vi "rad_Deploy Application Image.vi"(7 "App Image Temp Folder":path=path "C:/dev/Architectures/Reference Designs/Application Deployment and Replication/Application Deployment Utility/trunk/source/Application Images/_temp", 8 "error in (no error)":errorcluster, 10 "Selected Targets":T1[](array[typedef]) {"Primary NIC"."IP Address Request Mode" items=["Static"=1, "DHCP/Link-Local"=2, "Link-Local Only"=4, "DHCP Only"=8]}, 11 "App Image Path":path=path "C:/dev/Architectures/Reference Designs/Application Deployment and Replication/Application Deployment Utility/trunk/source/Application Images/AppImage1.lvappimg") -> (0 "error out":errorcluster, 1 "Cancelled":bool)   [LabVIEW 2023]
uses:
  Targets/TypeDefs/rad_Target Information.ctl
  Targets/TypeDefs/rad_Target Network Settings.ctl
  TypeDefs/rad_Target Configuration Settings.ctl
  TypeDefs/rad_Target Configuration Operations.ctl
  TypeDefs/rad_Deployment Notifiers.ctl
  TypeDefs/rad_Deployment Status Data Type.ctl
  TypeDefs/rad_Deployment Progress Data Type.ctl
  Util/FP Control/FP Control Functions.ctl
  <vilib>/nisyscfg/Close (System).vi
  <vilib>/nisyscfg/nisyscfg.lvlib
panel:
  out "Stop Updates":bool
  in  "Deploy":bool
  in  "Config Options":bool
  in  "Log":bool
  in  "Stop":bool
  in  "State Variables":T6={"App Image Path"=path "C:/dev/Architectures/Reference Designs/Application Deployment and Replication/Application Deployment Utility/trunk/source/Application Images/AppImage1.lvappimg", "App Image Temp Folder"=path "C:/dev/Architectures/Reference Designs/Application Deployment and Replication/Application Deployment Utility/trunk/source/Application Images/_temp", "Targets"=[], "Target Configuration Options"={"NumInBatch"=0, "Target Config Operation"=enum."No Config", "Target Name"="", "Increment Static IPs"=FALSE, "Change Target Name"=FALSE, "Primary NIC"={"MAC address"="", "IP Address Request Mode"=2, "IP address"="", "Subnet mask"="", "Gateway"="", "DNS server"=""}}, "Deployment Notifiers"=[]} {"Target Configuration Options"."Primary NIC"."IP Address Request Mode" items=["Static"=1, "DHCP/Link-Local"=2, "Link-Local Only"=4, "DHCP Only"=8]; "Targets"."Primary NIC"."IP Address Request Mode" items=["Static"=1, "DHCP/Link-Local"=2, "Link-Local Only"=4, "DHCP Only"=8]}
  out "Targets":i32(listbox)
  in  "Close":bool
  # "Targets"
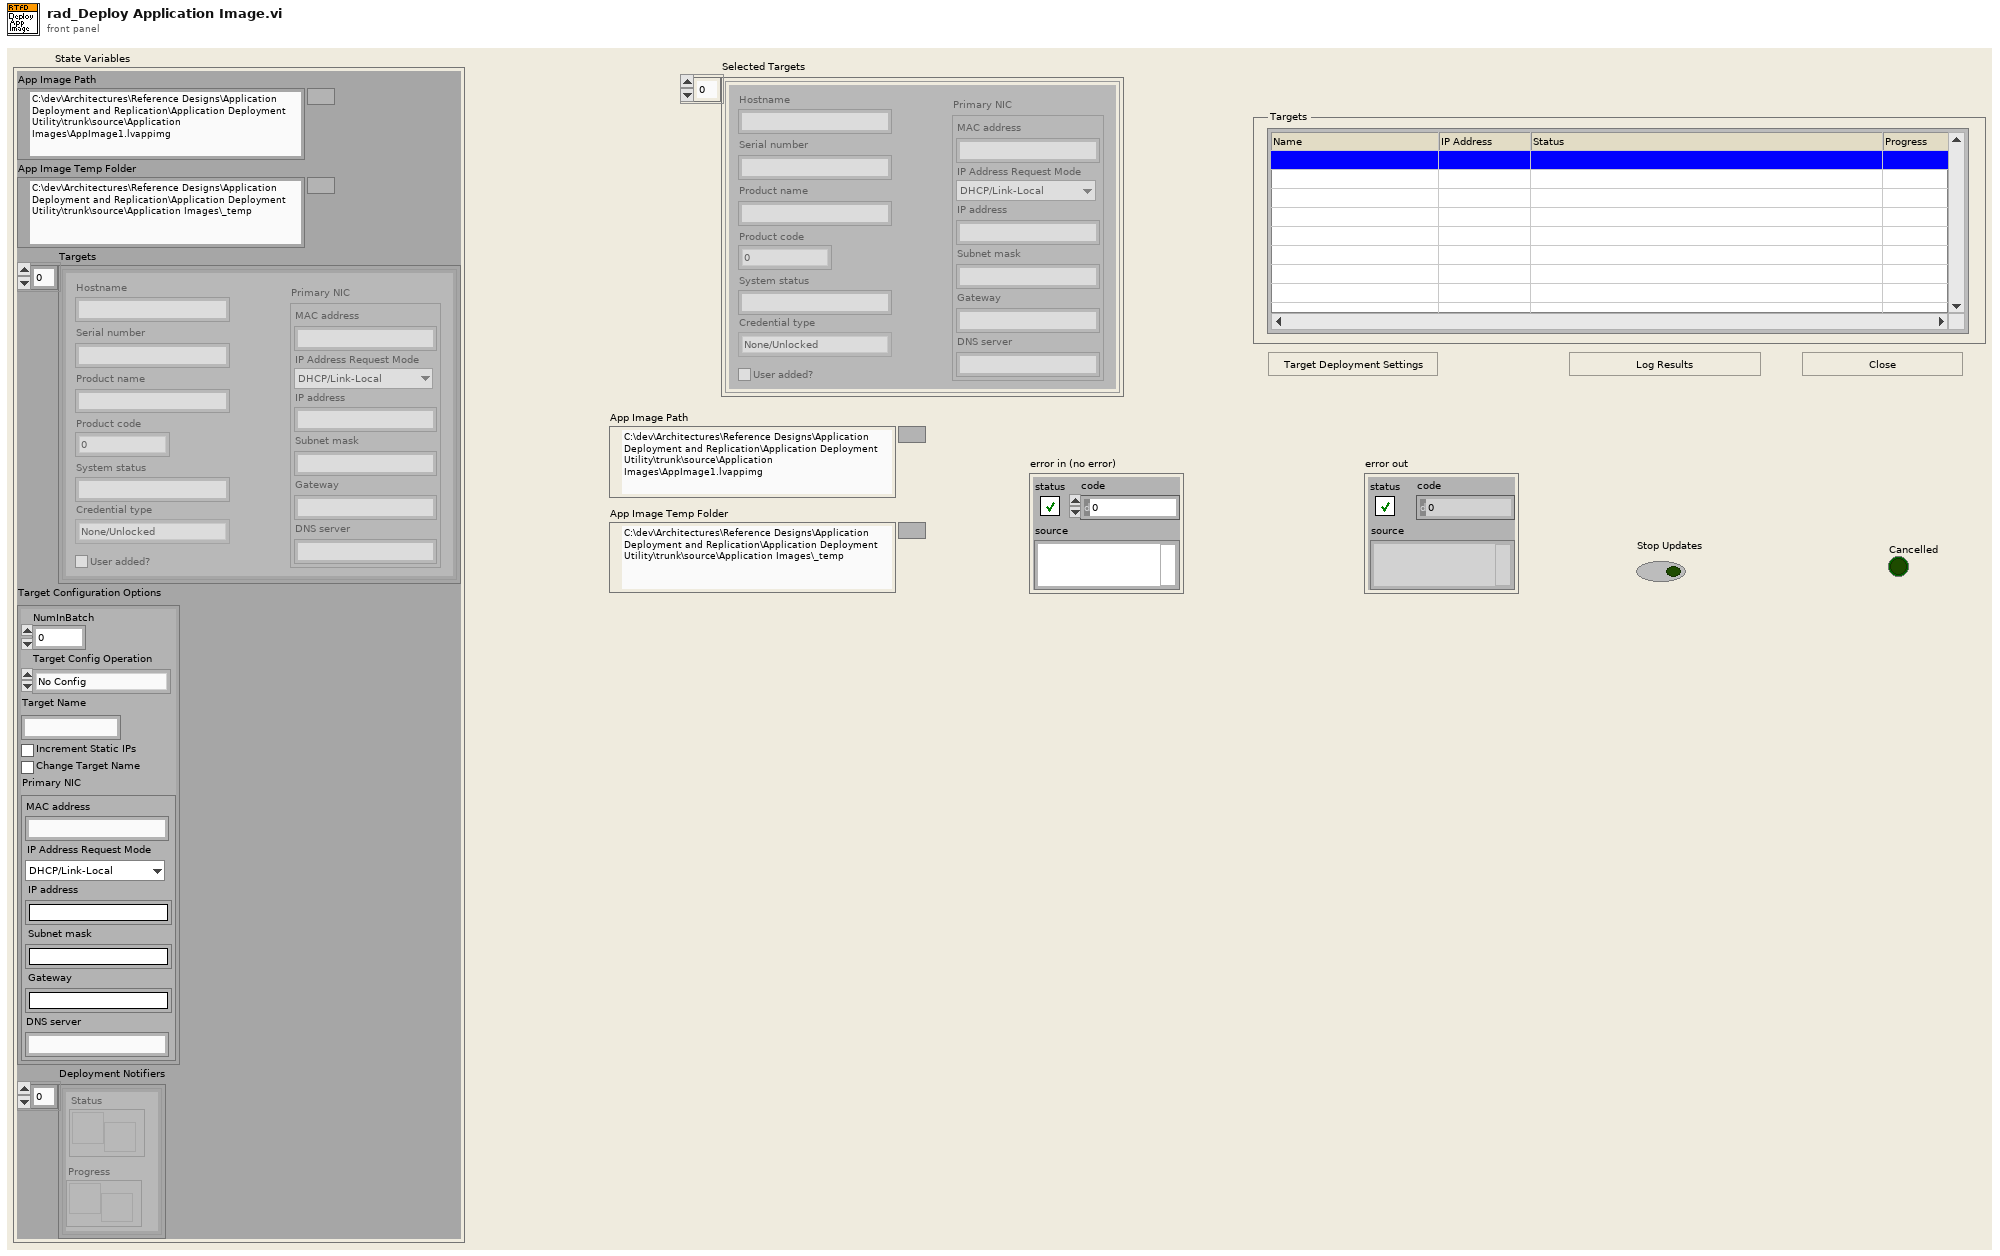
[diagram p1: front panel]
types:
  T1 = typedef "rad_Target Information.ctl" = cluster{"Hostname":string, "Serial number":string, "Product name":string, "Product code":i32, "System status":string, "Credential type":enum16{"None/Unlocked", "FTP Password", "NIAuth Credentials"}, "User added?":bool, "Primary NIC":T2}
  T2 = typedef "rad_Target Network Settings.ctl" = cluster{"MAC address":string, "IP Address Request Mode":i32, "IP address":string, "Subnet mask":string, "Gateway":string, "DNS server":string}
  T3 = typedef "rad_Target Configuration Settings.ctl" = cluster{"NumInBatch":u32, "Target Config Operation":T4, "Target Name":string, "Increment Static IPs":bool, "Change Target Name":bool, "Primary NIC":T2}
  T4 = typedef "rad_Target Configuration Operations.ctl" = enum8{"No Config", "Image Config", "Static Config"}
  T5 = typedef "rad_Deployment Notifiers.ctl" = cluster{"Status":refnum<notifier>, "Progress":refnum<notifier>}
  T6 = cluster{"App Image Path":path, "App Image Temp Folder":path, "Targets":T1[], "Target Configuration Options":T3, "Deployment Notifiers":T5[]}
  T7 = typedef "rad_Deployment Progress Data Type.ctl" = i8
  T8 = typedef "rad_Deployment Status Data Type.ctl" = string
  T9 = typedef "FP Control Functions.ctl" = enum16{"Open", "Close", "Bring To Front", "Center"}
  T10 = enum8{"Enabled", "Disabled", "Disabled and Grayed Out"}
  T11 = typedef "rad_Application Image Properties.ctl" = cluster{"Name":string, "Version":string, "Time":timestamp, "Description":string, "Key":string, "Chassis":string, "FPGA Properties":T12, "Model":string, "Retrieve":string[], "Deploy":string[], "Installed Software":string[]}
  T12 = typedef "rad_FPGA Properties.ctl" = T13[]
  T13 = typedef "rad_FPGA Flash Properties.ctl" = cluster{"Resource Name":string, "Path":path}
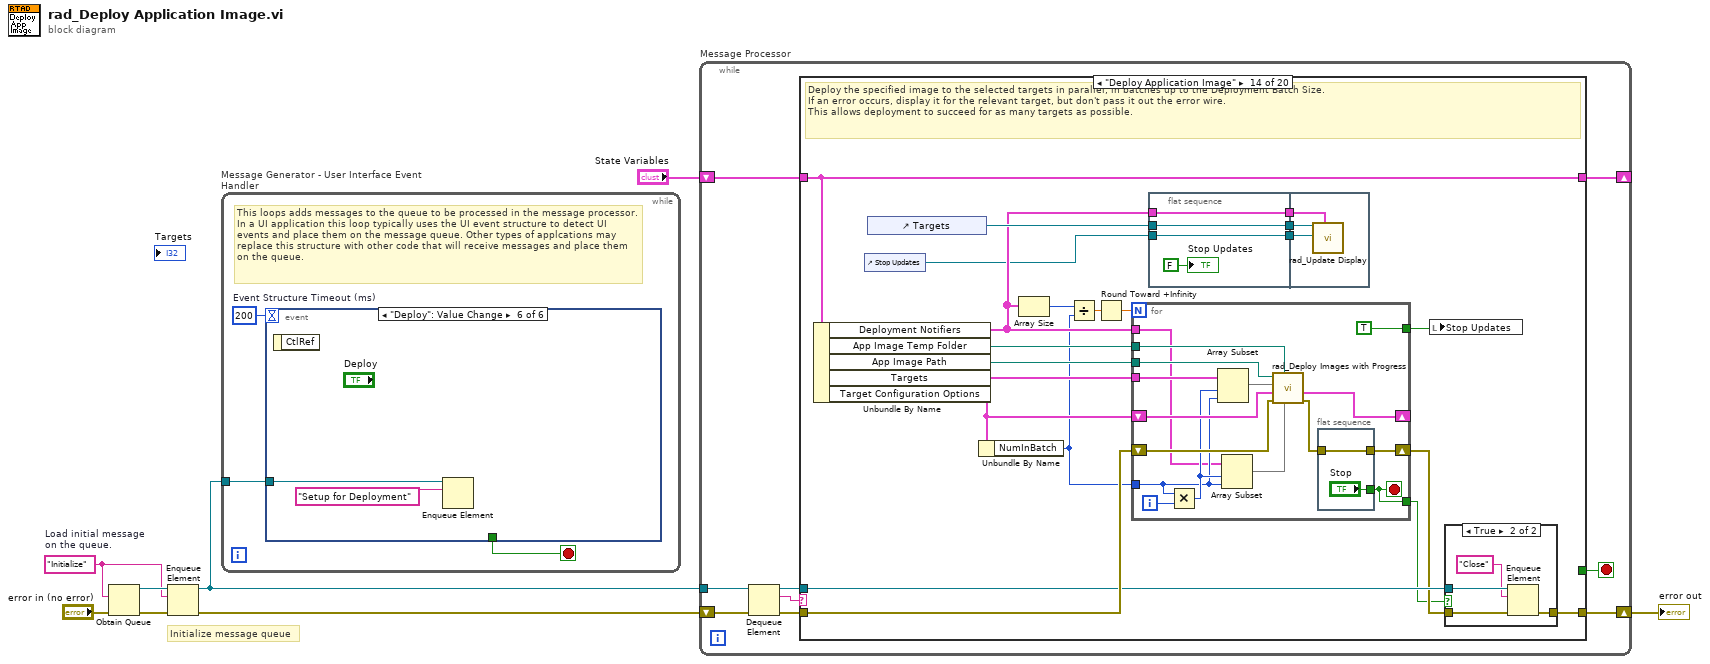
[diagram p0: block diagram]
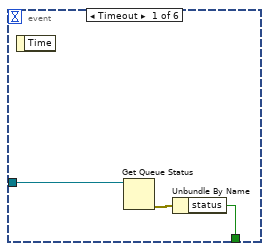
[diagram p2: hidden frame]
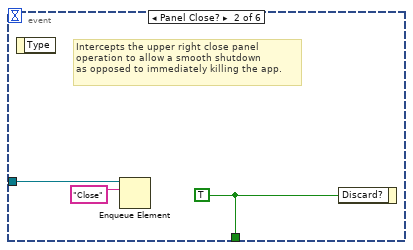
[diagram p3: hidden frame]
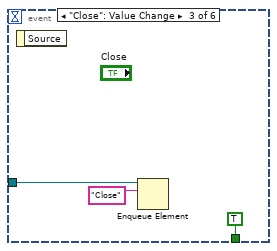
[diagram p4: hidden frame]
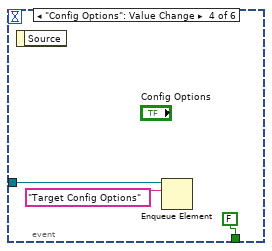
[diagram p5: hidden frame]
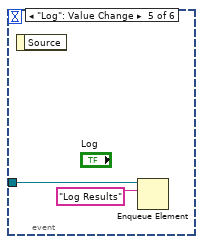
[diagram p6: hidden frame]
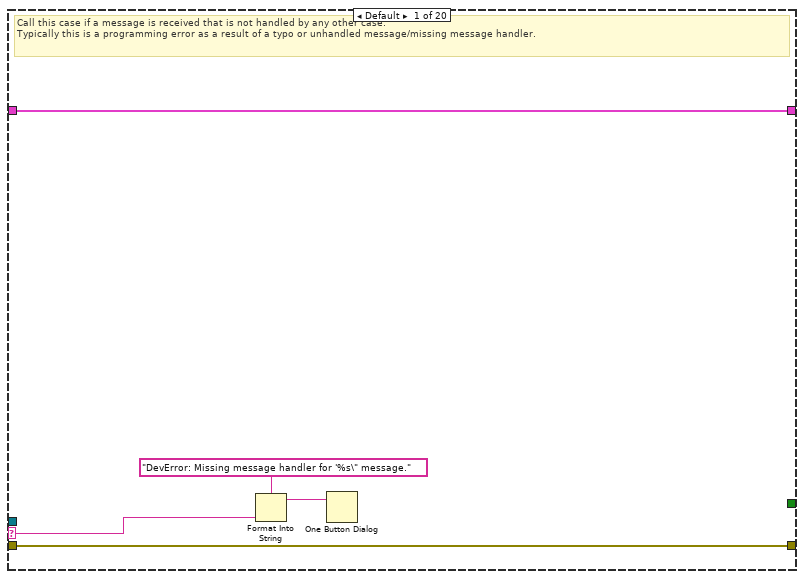
[diagram p7: hidden frame]
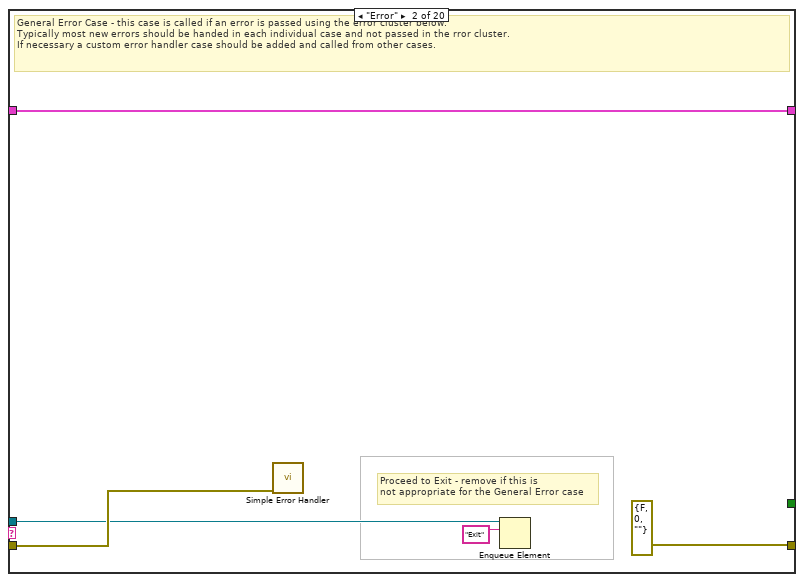
[diagram p8: hidden frame]
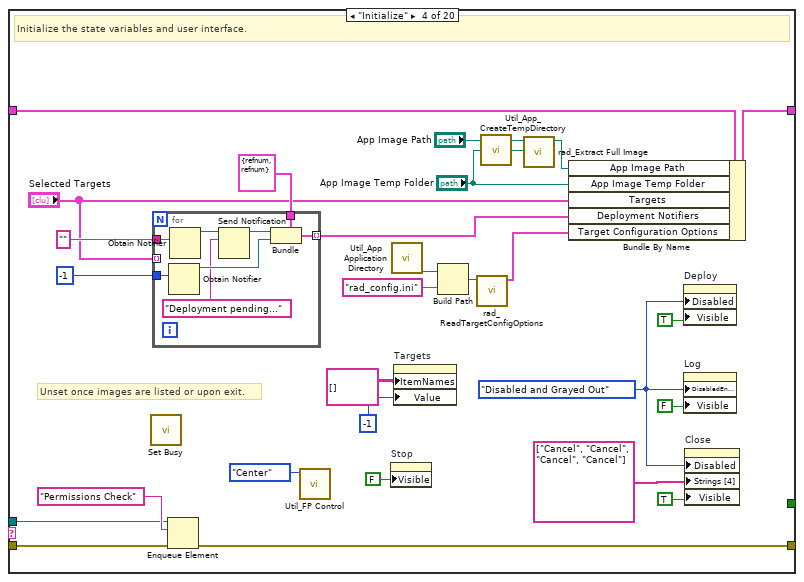
[diagram p10: hidden frame]
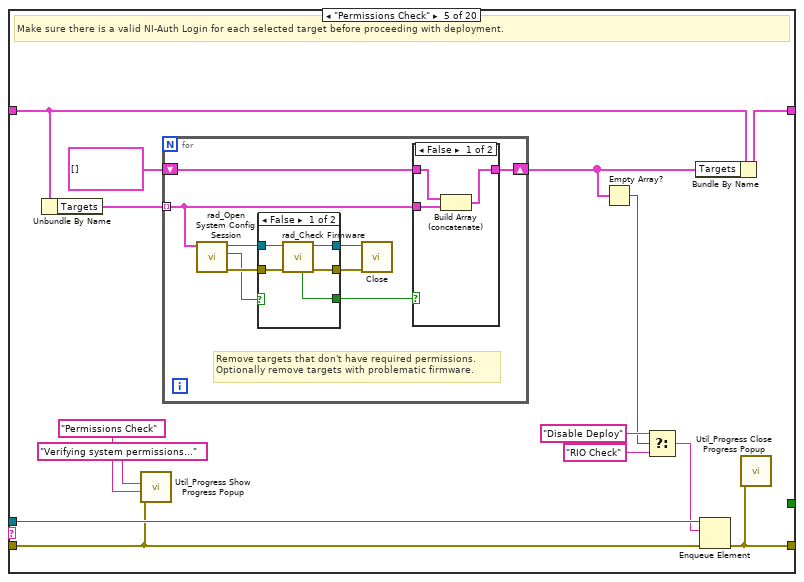
[diagram p11: hidden frame]
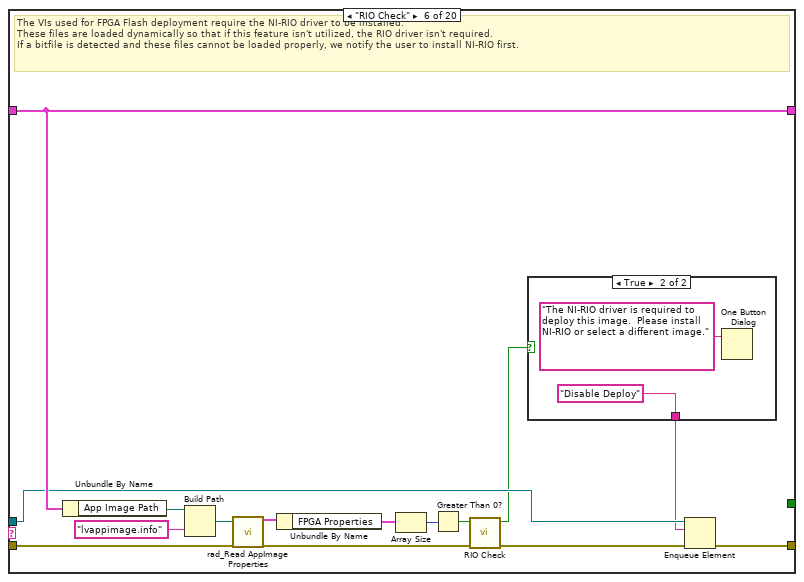
[diagram p14: hidden frame]
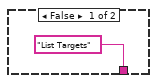
[diagram p15: hidden frame]
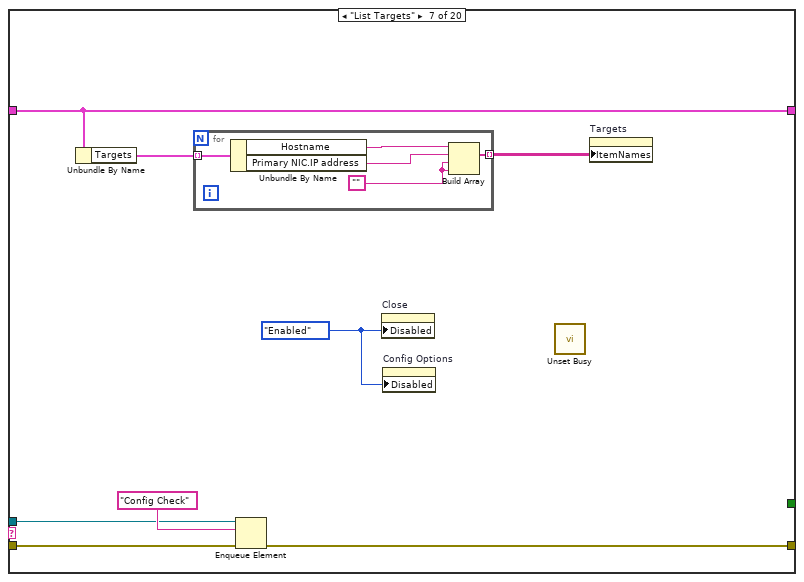
[diagram p16: hidden frame]
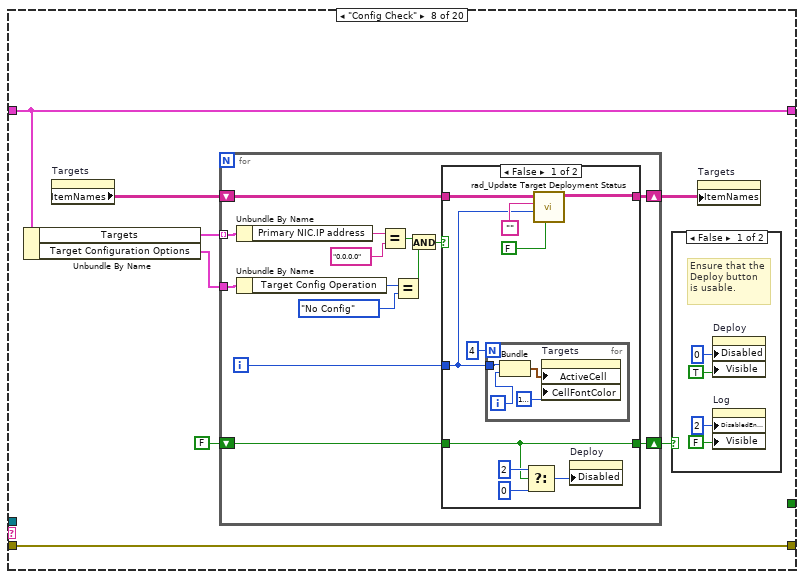
[diagram p17: hidden frame]
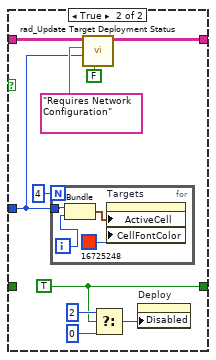
[diagram p19: hidden frame]
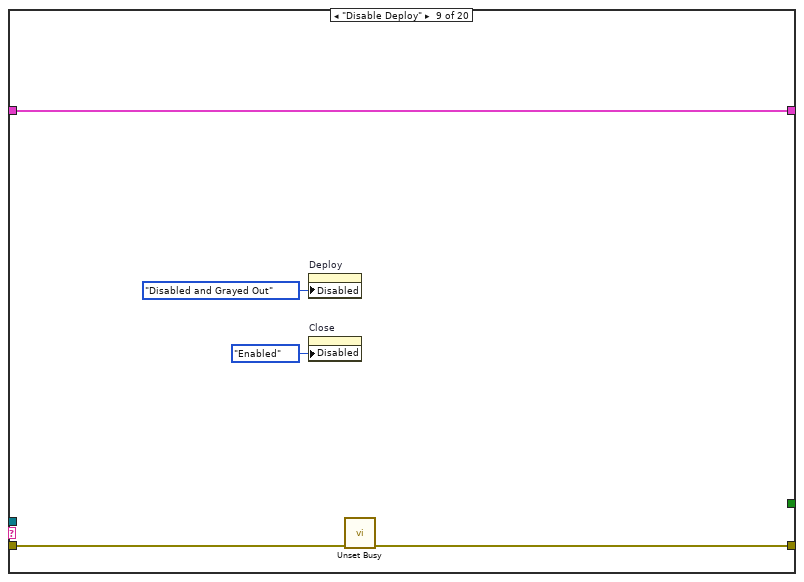
[diagram p20: hidden frame]
diagram:
  w1 = "Initialize"  # Load initial message on the queue.
  # "Initialize message queue"
  n1 = Obtain Queue(element data type=w1, error in (no error)="error in (no error)") -> (queue out=w3:refnum<queue>, error out=w8:errorcluster)  [unwired: 3 in, 1 out]
  n2 = Enqueue Element(queue=w3, element=w1, error in (no error)=w8) -> (queue out=w2:refnum<queue>, error out=w4:errorcluster)  [unwired: 1 in, 1 out]
  n3 = while "Message Generator - User Interface Event Handler" {
    tunnel: w2 -> [w9]
    stop <- w10 stop-if-true
    w11 = 200  # Event Structure Timeout (ms)
    # "This loops adds messages to the queue to be processed in the message processor. In a UI application this loop typically uses the UI event structure to detect UI events and place them on the message queue. Other types of applcations may replace this structure with other code that will receive messages and place them on the queue."
    n4 = event shown="[5] \"Deploy\": Value Change" {
      selector: _ -> [_ _ _ _ _ _]
      dyn-events: _ -> [_ _ _ _ _ _]
      timeout: w11 -> [_ _ _ _ _ _]
      tunnel: [w13 w17 TRUE ("Discard?") FALSE ("Discard?") _ _] -> w10
      tunnel: w9 -> [w12 w16 w20 w23 w25 w27]
      event Timeout {
        n5 = event-data() -> ()  [unwired: 2 out]
        n6 = Get Queue Status(queue=w12) -> (error out=w14:errorcluster)  [unwired: 2 in, 7 out]
        n7 = Unbundle By Name(w14) -> ("status"=w13:bool)
      }
      event Panel Close? {
        w17 = TRUE ("Discard?")
        # "Intercepts the upper right close panel\noperation to allow a smooth shutdown\nas opposed to immediately killing the app."
        n8 = event-data() -> ()  [unwired: 2 out]
        n9 = Enqueue Element(queue=w16, element="Close") -> ()  [unwired: 2 in, 3 out]
        n10 = event-data("Discard?"=w17) -> ()  [unwired: 1 in, 1 out]
      }
      event "Close": Value Change {
        n11 = event-data() -> ()  [unwired: 2 out]
        n12 = Enqueue Element(queue=w20, element="Close") -> ()  [unwired: 2 in, 3 out]
      }
      event "Config Options": Value Change {
        n13 = event-data() -> ()  [unwired: 2 out]
        n14 = Enqueue Element(queue=w23, element="Target Config Options") -> ()  [unwired: 2 in, 3 out]
      }
      event "Log": Value Change {
        n15 = event-data() -> ()  [unwired: 2 out]
        n16 = Enqueue Element(queue=w25, element="Log Results") -> ()  [unwired: 2 in, 3 out]
      }
      event "Deploy": Value Change {
        n17 = event-data() -> ()  [unwired: 2 out]
        n18 = Enqueue Element(queue=w27, element="Setup for Deployment") -> ()  [unwired: 2 in, 3 out]
      }
    }
  }
  n19 = while "Message Processor" {
    shift-left: w4 -> [w31]
    shift-right: [w32] -> w5
    tunnel: w2 -> [w30]
    shift-left: "State Variables" -> [w36]
    shift-right: [w35] -> _
    stop <- w28 stop-if-true
    n20 = Dequeue Element(queue=w30, error in (no error)=w31) -> (queue out=w34:refnum<queue>, element=w29:string, error out=w33:errorcluster)  [unwired: 1 in, 1 out]
    n21 = case shown="\"Deploy Application Image\"" w29 {
      selector: w29 -> [w39 _ _ _ _ _ _ _ _ _ _ _ _ _ _ _ _ _ _ _]
      tunnel: [w41 w46 w48 w75 w95 w131 w143 w153 w207 w211 w213 w219 w239 w258 w295 w303 w305 w313 w316 w323] -> w35
      tunnel: w36 -> [w41 w46 w48 w76 w96 w131 w143 w153 w207 w211 w213 w220 w239 w258 w295 w303 w305 w313 w316 w323]
      tunnel: w34 -> [_ w43 _ w54 w94 w128 w138 _ _ _ _ w217 w235 w253 _ _ _ w307 _ w328]
      tunnel: w33 -> [w40 w44 w47 w70 w90 w123 w140 w158 w209 w210 w212 w221 w240 w257 w296 w301 w304 w308 w314 w329]
      tunnel: [w40 errorcluster {"status"=FALSE, "code"=0, "source"=""} ("error out") w47 w56 w89 w129 w139 w158 w208 w210 w212 w215 w231 w251 w296 w300 w304 w306 w314 w320] -> w32
      tunnel: [_ _ _ _ _ _ _ _ _ _ _ _ _ _ _ _ _ _ _ TRUE] -> w28
      frame Default {
        # "Call this case if a message is received that is not handled by any other case.\nTypically this is a programming error as a result of a typo or unhandled message/missing message handler."
        n22 = Format Into String(format string="DevError: Missing message handler for '%s\" message." ("message"), w39) -> (resulting string=w37:string)  [unwired: 2 in, 1 out]
        n23 = One Button Dialog(message=w37) -> ()  [unwired: 2 out]
      }
      frame "Error" {
        # "Proceed to Exit - remove if this is\nnot appropriate for the General Error case"
        # "General Error Case - this case is called if an error is passed using the error cluster below.\nTypically most new errors should be handed in each individual case and not passed in the rror cluster.\nIf necessary a custom error handler case should be added and called from other cases."
        n24 = call <vilib>:"Simple Error Handler.vi"("error in (no error)"=w44) -> ()  [unwired: 1 in, 8 out]
        n25 = Enqueue Element(queue=w43, element="Exit") -> ()  [unwired: 2 in, 3 out]
      }
      frame "*******Init******" {
        # "Dummy case to add a seperator in the Case Structure menu."
      }
      frame "Initialize" {
        w49 = T10."Disabled and Grayed Out" ("Disabled")
        # "Unset once images are listed or upon exit."
        # "Initialize the state variables and user interface."
        n26 = call <vilib>:"Set Busy.vi"() -> ()  [unwired: 10 in, 2 out]
        n27 = for {
          tunnel: T8 "" ("status notifier data type") -> [w84]
          tunnel: T7 -1 ("Progress") -> [w83]
          tunnel: T5 {"Status"=refnum, "Progress"=refnum} ("Deployment Notifiers") -> [w81]
          tunnel: [w80] -> w65 mode=indexing
          tunnel: "Selected Targets" -> [_] mode=indexing
          n28 = Obtain Notifier(notification data type=w83) -> (notifier out=w82:refnum<notifier>)  [unwired: 3 in, 2 out]
          n29 = Obtain Notifier(notification data type=w84) -> (notifier out=w79:refnum<notifier>)  [unwired: 3 in, 2 out]
          n30 = Send Notification(notification=T8 "Deployment pending...", notifier=w79) -> (notifier out=w78:refnum<notifier>)  [unwired: 1 in, 1 out]
          n31 = Bundle(cluster=w81, "Status"=w78, "Progress"=w82) -> (w80:T5)
        }
        n32 = Enqueue Element(queue=w54, element="Permissions Check", error in (no error)=w70) -> (error out=w56:errorcluster)  [unwired: 1 in, 2 out]
        n33 = call "Util_FP Control.vi"("Function"=FP_Control_Functions."Center") -> ()  [unwired: 1 in, 10 out]
        n34 = property on="Stop" class="Bool"("Visible"=FALSE) -> ()  [unwired: 2 in, 2 out]
        n35 = call "Util_App Application Directory.vi"() -> ("Application Directory"=w64:path)  [unwired: 11 out]
        n36 = property on="Targets" class="MCListbox (strict)"("ItemNames"=string[][] [] ("Item Names"), "Value"=-1 ("Targets")) -> ()  [unwired: 2 in, 2 out]
        n37 = Build Path(base path=w64, name or relative path="rad_config.ini" ("Config File Name")) -> (appended path=w62:path)
        n38 = call "rad_ReadTargetConfigOptions.vi"("configuration file path"=w62) -> ("TargetConfigurationOptions"=w61:T3)  [unwired: 9 in, 1 out]
        n39 = call "Util_App_CreateTempDirectory.vi"("TempFolderPath"="App Image Temp Folder") -> ("TempFolderPath_out"=w58:path)
        n40 = call "rad_Extract Full Image.vi"("App Image Temp Folder"=w58, "Zipped App Image File Path"="App Image Path") -> ("Unzipped App Image Folder Path"=w59:path)  [unwired: 8 in, 1 out]
        n41 = Bundle By Name(cluster=w76, "App Image Path"=w59, "App Image Temp Folder"="App Image Temp Folder", "Targets"="Selected Targets", "Deployment Notifiers"=w65, "Target Configuration Options"=w61) -> (w75:T6)
        n42 = property on="Deploy" class="Bool"("Disabled"=w49, "Visible"=TRUE) -> ()  [unwired: 2 in, 2 out]
        n43 = property on="Log" class="Bool"("DisabledEnum"=w49, "Visible"=FALSE) -> ()  [unwired: 2 in, 2 out]
        n44 = property on="Close" class="Bool"("Disabled"=w49, "Strings [4]"=string[] ["Cancel", "Cancel", "Cancel", "Cancel"], "Visible"=TRUE) -> ()  [unwired: 2 in, 2 out]
      }
      frame "Permissions Check" {
        # "Make sure there is a valid NI-Auth Login for each selected target before proceeding with deployment."
        n45 = Unbundle By Name(w96) -> ("Targets"=w98:T1[])
        n46 = call "Util_Progress Show Progress Popup.vi"("error in (no error)"=w90, "Title"="Permissions Check" ("Message"), "Message"="Verifying system permissions...") -> ()  [unwired: 8 in, 1 out]
        n47 = for {
          tunnel: w98 -> [w105] mode=indexing
          shift-right: [w107] -> w86
          shift-left: T1[] [] -> [w106]
          # "Remove targets that don't have required permissions.\nOptionally remove targets with problematic firmware."
          n48 = call "rad_Open System Config Session.vi"("Target settings"=w105) -> ("error out"=w104:errorcluster, "Cancelled"=w99:bool, "Session out"=w102:refnum<k21>)  [unwired: 7 in, 1 out]
          n49 = case shown="False" w99 {
            selector: w99 -> [_ w113]
            tunnel: w104 -> [w112 w115]
            tunnel: [w109 w115] -> w103
            tunnel: w102 -> [w111 w114]
            tunnel: [w110 w114] -> w101
            tunnel: [w108 w113] -> w100
            frame False {
              n50 = call "rad_Check Firmware.vi"("error in (no error)"=w112, "System Configuration"=w111) -> ("error out"=w109:errorcluster, "System Configuration out"=w110:refnum<k21>, "Bad firmware and user canceled"=w108:bool)  [unwired: 7 in]
            }
            frame True {
            }
          }
          n51 = call-poly <vilib>:"Close.vi"("error in (no error)"=w103, "Session in"=w101) -> ()  [unwired: 9 in, 1 out]
          n52 = case shown="False" w100 {
            tunnel: w105 -> [w118 _]
            tunnel: [w117 w119] -> w107
            tunnel: w106 -> [w116 w119]
            frame False {
              n53 = Build Array (concatenate)(w116, w118) -> (w117:T1[])
            }
            frame True {
            }
          }
        }
        n54 = Empty Array?(array=w86) -> (empty?=w85:bool)
        n55 = Select(t="Disable Deploy", s=w85, f="RIO Check") -> (s? t:f=w91:string)
        n56 = Bundle By Name(cluster=w96, "Targets"=w86) -> (w95:T6)
        n57 = Enqueue Element(queue=w94, element=w91, error in (no error)=w90) -> (error out=w89:errorcluster)  [unwired: 1 in, 2 out]
        n58 = call "Util_Progress Close Progress Popup.vi"("error in (no error)"=w89) -> ()  [unwired: 10 in, 1 out]
      }
      frame "RIO Check" {
        # "The VIs used for FPGA Flash deployment require the NI-RIO driver to be installed.  \nThese files are loaded dynamically so that if this feature isn't utilized, the RIO driver isn't required.\nIf a bitfile is detected and these files cannot be loaded properly, we notify the user to install NI-RIO first."
        n59 = Unbundle By Name(w131) -> ("App Image Path"=w121:path)
        n60 = Build Path(base path=w121, name or relative path="lvappimage.info") -> (appended path=w120:path)
        n61 = call "rad_Read AppImage Properties.vi"("AppImage Properties Path"=w120, "error in (no error)"=w123) -> ("AppImage Properties"=w124:T11, "error out"=w125:errorcluster)  [unwired: 12 in, 4 out]
        n62 = Unbundle By Name(w124) -> ("FPGA Properties"=w134:T12)
        n63 = Array Size(array=w134) -> (size(s)=w133:i32)
        n64 = Greater Than 0?(x=w133) -> (x > 0?=w132:bool)
        n65 = call "RIO Check.vi"("error in"=w125, "Requires RIO"=w132) -> ("error out"=w130:errorcluster, "RIO needed but not installed"=w127:bool)  [unwired: 8 in]
        n66 = case shown="True" w127 {
          tunnel: ["List Targets" "Disable Deploy" ("t")] -> w126
          frame False {
          }
          frame True {
            n67 = One Button Dialog(message="The NI-RIO driver is required to deploy this image.  Please install NI-RIO or select a different image.") -> ()  [unwired: 1 in, 1 out]
          }
        }
        n68 = Enqueue Element(queue=w128, element=w126, error in (no error)=w130) -> (error out=w129:errorcluster)  [unwired: 1 in, 2 out]
      }
      frame "List Targets" {
        w142 = T10."Enabled" ("Disabled")
        n69 = Unbundle By Name(w143) -> ("Targets"=w145:T1[])
        n70 = for {
          tunnel: w145 -> [w150] mode=indexing
          tunnel: [w147] -> w144 mode=indexing
          w146 = ""
          n71 = Unbundle By Name(w150) -> ("Hostname"=w149:string, "Primary NIC.IP address"=w148:string)
          n72 = Build Array(w149, w148, w146, w146) -> (w147:string[])
        }
        n73 = Enqueue Element(queue=w138, element="Config Check", error in (no error)=w140) -> (error out=w139:errorcluster)  [unwired: 1 in, 2 out]
        n74 = property on="Close" class="Bool"("Disabled"=w142) -> ()  [unwired: 2 in, 2 out]
        n75 = property on="Config Options" class="Bool"("Disabled"=w142) -> ()  [unwired: 2 in, 2 out]
        n76 = call <vilib>:"Unset Busy.vi"() -> ()  [unwired: 11 in, 1 out]
        n77 = property on="Targets" class="MCListbox (strict)"("ItemNames"=w144) -> ()  [unwired: 2 in, 2 out]
      }
      frame "Config Check" {
        n78 = Unbundle By Name(w153) -> ("Targets"=w156:T1[], "Target Configuration Options"=w157:T3)
        n79 = property on="Targets" class="MCListbox (strict)"() -> ("ItemNames"=w152:string[][])  [unwired: 2 in, 2 out]
        n80 = for {
          tunnel: w156 -> [w167] mode=indexing
          tunnel: w157 -> [w166]
          shift-right: [w163] -> w151
          shift-left: FALSE -> [w164]
          shift-right: [w169] -> w154
          shift-left: w152 -> [w165]
          i -> [w168]
          n81 = Unbundle By Name(w167) -> ("Primary NIC.IP address"=w176:string)
          n82 = Unbundle By Name(w166) -> ("Target Config Operation"=w174:T4)
          n83 = Equal?(x=w176, y="0.0.0.0") -> (x = y?=w172:bool)
          n84 = Equal?(x=w174, y=rad_Target_Configuration_Operations."No Config") -> (x = y?=w170:bool)
          n85 = And(x=w172, y=w170) -> (x .and. y?=w171:bool)
          n86 = case shown="False" w171 {
            tunnel: [w185 w200] -> w169
            tunnel: w168 -> [w183 w196]
            tunnel: w165 -> [w186 w197]
            tunnel: w164 -> [w178 _]
            tunnel: [w178 w193] -> w163
            frame False {
              n87 = for {
                N: 4 -> [_]
                tunnel: w183 -> [w189]
                i -> [w188]
                n88 = Bundle(w189, w188) -> (w187:cluster{i32, i32})  [unwired: 1 in]
                n89 = property on="Targets" class="MCListbox (strict)"("ActiveCell"=w187, "CellFontColor"=u32 16777222) -> ()  [unwired: 2 in, 2 out]
              }
              n90 = Select(t=2, s=w178, f=0) -> (s? t:f=w179:i32)
              n91 = call "rad_Update Target Deployment Status.vi"("Add Timestamp?"=FALSE, "Target Index"=w183, "Message"="", "Targets Deployment Status"=w186) -> ("Targets Deployment Status"=w185:string[][])  [unwired: 7 in]
              n92 = property on="Deploy" class="Bool"("Disabled"=w179) -> ()  [unwired: 2 in, 2 out]
            }
            frame True {
              w193 = TRUE
              n93 = for {
                N: 4 -> [_]
                tunnel: w196 -> [w203]
                i -> [w202]
                n94 = Bundle(w203, w202) -> (w201:cluster{i32, i32})  [unwired: 1 in]
                n95 = property on="Targets" class="MCListbox (strict)"("ActiveCell"=w201, "CellFontColor"=u32 16725248) -> ()  [unwired: 2 in, 2 out]
              }
              n96 = call "rad_Update Target Deployment Status.vi"("Add Timestamp?"=FALSE, "Target Index"=w196, "Message"="Requires Network Configuration", "Targets Deployment Status"=w197) -> ("Targets Deployment Status"=w200:string[][])  [unwired: 7 in]
              n97 = Select(t=2, s=w193, f=0) -> (s? t:f=w192:i32)
              n98 = property on="Deploy" class="Bool"("Disabled"=w192) -> ()  [unwired: 2 in, 2 out]
            }
          }
        }
        n99 = case shown="False" w151 {
          frame False {
            # "Ensure that the\nDeploy button\nis usable."
            n100 = property on="Deploy" class="Bool"("Disabled"=0, "Visible"=TRUE) -> ()  [unwired: 2 in, 2 out]
            n101 = property on="Log" class="Bool"("DisabledEnum"=2, "Visible"=FALSE) -> ()  [unwired: 2 in, 2 out]
          }
          frame True {
          }
        }
        n102 = property on="Targets" class="MCListbox (strict)"("ItemNames"=w154) -> ()  [unwired: 2 in, 2 out]
      }
      frame "Disable Deploy" {
        n103 = property on="Deploy" class="Bool"("Disabled"=T10."Disabled and Grayed Out") -> ()  [unwired: 2 in, 2 out]
        n104 = property on="Close" class="Bool"("Disabled"=T10."Enabled") -> ()  [unwired: 2 in, 2 out]
        n105 = call <vilib>:"Unset Busy.vi"("error in (no error)"=w209) -> ("error out"=w208:errorcluster)  [unwired: 10 in]
      }
      frame "*****************" {
        # "Dummy case to add a seperator in the Case Structure menu."
      }
      frame "Update Display" {
      }
      frame "Target Config Options" {
        # "Update the options for the network configuration settings which may be applied to each RT target after deploying the application image."
        n106 = Unbundle By Name(w220) -> ("Target Configuration Options"=w222:T3)
        n107 = call "rad_Target Configuration Options Dialog.vi"("error in"=w221, "Target Configuration Options"=w222) -> ("error out"=w216:errorcluster, "Cancelled"=w214:bool, "Target Configuration Options"=w218:T3)  [unwired: 7 in]
        n108 = case shown="False" w214 {
          tunnel: w217 -> [w226 _]
          tunnel: w216 -> [w225 w227]
          tunnel: [w224 w227] -> w215
          frame False {
            n109 = Enqueue Element(queue=w226, element="Config Check" ("Message Name"), error in (no error)=w225) -> (error out=w224:errorcluster)  [unwired: 1 in, 2 out]
          }
          frame True {
          }
        }
        n110 = Bundle By Name(cluster=w220, "Target Configuration Options"=w218) -> (w219:T6)
      }
      frame "Setup for Deployment" {
        w237 = T10."Disabled and Grayed Out" ("Disabled")
        # "Update the UI for the deployment process - disable some buttons."
        n111 = Enqueue Element(queue=w235, element="Deploy Application Image", error in (no error)=w240) -> (queue out=w232:refnum<queue>, error out=w233:errorcluster)  [unwired: 1 in, 1 out]
        n112 = property on="Stop" class="Bool"("Visible"=TRUE) -> ()  [unwired: 2 in, 2 out]
        n113 = property on="Close" class="Bool"("Disabled"=w237, "Visible"=FALSE) -> ()  [unwired: 2 in, 2 out]
        n114 = property on="Config Options" class="Bool"("Disabled"=w237) -> ()  [unwired: 2 in, 2 out]
        n115 = property on="Log" class="Bool"("Disabled"=w237, "Visible"=TRUE) -> ()  [unwired: 2 in, 2 out]
        n116 = Enqueue Element(queue=w232, element="Cleanup from Deployment", error in (no error)=w233) -> (error out=w231:errorcluster)  [unwired: 1 in, 2 out]
        n117 = property on="Deploy" class="Bool"("Visible"=FALSE) -> ()  [unwired: 2 in, 2 out]
      }
      frame "Deploy Application Image" {
        # "Deploy the specified image to the selected targets in parallel, in batches up to the Deployment Batch Size.\nIf an error occurs, display it for the relevant target, but don't pass it out the error wire.\nThis allows deployment to succeed for as many targets as possible."
        n118 = Unbundle By Name(w258) -> ("Deployment Notifiers"=w248:T5[], "App Image Temp Folder"=w259:path, "App Image Path"=w261:path, "Targets"=w260:T1[], "Target Configuration Options"=w242:T3)
        n119 = control-ref of="Stop Updates"() -> (w244:refnum<vi>)
        n120 = control-ref of="Targets"() -> (w249:refnum<vi>)
        n121 = Unbundle By Name(w242) -> ("NumInBatch"=w241:u32)
        n122 = Array Size(array=w248) -> (size(s)=w256:i32)
        n123 = Divide(x=w256, y=w241) -> (x/y=w255:dbl)
        n124 = Round Toward +Infinity(x=w255) -> (ceil(x): smallest int >= x=w254:dbl)
        n125 = for {
          N: w254 -> [_]
          tunnel: w261 -> [w288]
          tunnel: w260 -> [w283]
          tunnel: w259 -> [w287]
          tunnel: w241 -> [w280]
          shift-right: [w279] -> w252
          shift-left: w257 -> [w286]
          tunnel: [w277] -> w250
          tunnel: w248 -> [w276]
          tunnel: [TRUE] -> w247
          shift-right: [w274] -> _
          shift-left: w242 -> [w289]
          i -> [w285]
          stop <- w277 stop-if-true
          n126 = Multiply(x=w280, y=w285) -> (x*y=w281:u32)
          n127 = Array Subset(array=w283, index=w281, length=w280) -> (w282:T1[])
          n128 = Array Subset(array=w276, index=w281, length=w280) -> (w284:T5[])
          n129 = call "rad_Deploy Images with Progress.vi"("Deployment Notifiers"=w284, "temp folder"=w287, "error in (no error)"=w286, "Target Config Options in"=w289, "RT Deployment Targets in"=w282, "image path"=w288) -> ("error out"=w278:errorcluster, "Target Config Options out"=w274:T3)  [unwired: 3 in, 1 out]
          n130 = flat-sequence {
            tunnel: ["Stop"] -> w277
            tunnel: [w290] -> w279
            tunnel: w278 -> [w290]
            frame #0 {
            }
          }
        }
        n131 = flat-sequence {
          tunnel: w248 -> [w264]
          tunnel: w249 -> [w265]
          tunnel: [w265] -> w246
          tunnel: [w264] -> w245
          tunnel: w244 -> [w263]
          tunnel: [w263] -> w243
          tunnel: w246 -> [w268]
          tunnel: w245 -> [w267]
          tunnel: w243 -> [w266]
          frame #0 {
            "Stop Updates" <- FALSE ("Stop Updates")
          }
          frame #1 {
            n132 = call "rad_Update Display.vi"("Deployment Notifiers"=w267, "Stop Updates"=w266, "Listbox Reference"=w268) -> ()  [unwired: 9 in]
          }
        }
        n133 = local write "Stop Updates"(w247) -> ()
        n134 = case shown="True" w250 {
          tunnel: w253 -> [_ w273]
          tunnel: w252 -> [w269 w272]
          tunnel: [w269 w271] -> w251
          frame False {
          }
          frame True {
            n135 = Enqueue Element(queue=w273, element="Close" ("Message Name"), error in (no error)=w272) -> (error out=w271:errorcluster)  [unwired: 1 in, 2 out]
          }
        }
      }
      frame "Cleanup from Deployment" {
        w293 = T10."Enabled" ("Disabled")
        # "Reset the UI after the deployment process."
        n136 = property on="Config Options" class="Bool"("Disabled"=w293) -> ()  [unwired: 2 in, 2 out]
        n137 = property on="Log" class="Bool"("Disabled"=w293) -> ()  [unwired: 2 in, 2 out]
        n138 = property on="Stop" class="Bool"("Visible"=FALSE) -> ()  [unwired: 2 in, 2 out]
        n139 = property on="Close" class="Bool"("Disabled"=w293, "Strings [4]"=string[] ["Close", "Close", "Close", "Close"], "Visible"=TRUE) -> ()  [unwired: 2 in, 2 out]
      }
      frame "Log Results" {
        # "Log the deployment information and results to a TSV file."
        n140 = Unbundle By Name(w303) -> ("Targets"=w302:T1[], "App Image Path"=w299:path)
        n141 = property on="Targets" class="MCListbox (strict)"() -> ("ItemNames"=w298:string[][])  [unwired: 2 in, 2 out]
        n142 = call "rad_Write Deployment Results to File.vi"("error in"=w301, "App Image Path"=w299, "Targets Deployment"=w298, "Targets"=w302) -> ("error out"=w300:errorcluster)  [unwired: 1 in, 6 out]
      }
      frame "******Close******" {
        # "Dummy case to add a seperator in the Case Structure menu."
      }
      frame "Close" {
        n143 = Enqueue Element(queue=w307, element="Cleanup Temp App Image", error in (no error)=w308) -> (queue out=w310:refnum<queue>, error out=w311:errorcluster)  [unwired: 1 in, 1 out]
        n144 = Enqueue Element(queue=w310, element="Exit", error in (no error)=w311) -> (error out=w306:errorcluster)  [unwired: 1 in, 2 out]
      }
      frame "Cleanup Temp App Image" {
        # "Empty the temp folder used during deployment."
        n145 = Unbundle By Name(w316) -> ("App Image Temp Folder"=w315:path)
        n146 = Delete(path (use dialog)=w315, entire hierarchy (F)=TRUE) -> ()  [unwired: 1 in, 5 out]
      }
      frame "Exit" {
        n147 = Unbundle By Name(w323) -> ("Deployment Notifiers"=w322:T5[])
        n148 = Release Queue(queue=w328, force destroy? (F)=TRUE, error in (no error)=w329) -> (error out=w321:errorcluster)  [unwired: 2 out]
        n149 = for {
          tunnel: w322 -> [w335] mode=indexing
          shift-right: [w330] -> w320
          shift-left: w321 -> [w333]
          n150 = Unbundle By Name(w335) -> ("Status"=w334:refnum<notifier>, "Progress"=w332:refnum<notifier>)
          n151 = Release Notifier(notifier=w334, force destroy? (F)=TRUE, error in (no error)=w333) -> (error out=w331:errorcluster)  [unwired: 2 out]
          n152 = Release Notifier(notifier=w332, force destroy? (F)=TRUE, error in (no error)=w331) -> (error out=w330:errorcluster)  [unwired: 2 out]
        }
        n153 = property on="Close" class="Bool"() -> ("Strings [4]"=w327:string[])  [unwired: 2 in, 2 out]
        n154 = Index Array(array=w327) -> (element=w326:string)  [unwired: 1 in]
        n155 = Equal?(x="Cancel", y=w326) -> (x = y?=→"Cancelled":bool)
        n156 = call <vilib>:"Unset Busy.vi"() -> ()  [unwired: 11 in, 1 out]
      }
    }
  }
  "error out" <- w5
